vi "ShotLogSave.vi"(10 "Experiment State":T1={"error"={"status"=FALSE, "code"=0, "source"=""}, "Digitizer DAQmx Tasks"={"TaskArray"=[]}, "Digitizer Settings"={"Channel Settings"=[], "Card Settings"=[]}, "Synchronization Settings"={"Synchronizer"="PXI1Slot2", "source terminal"="GlobalSoftwareTrigger"}, "Digitizer Data"=[], "Next Shot#"="0", "System Message"="", "User Shot Notes"="", "Timing Settings"={"Timing Card Settings"=[], "Timing Channel Settings"=[[{"Delay (s)"=2.559999942779541, "Pulse width (s)"=0.009999999776482582, "Active"=TRUE, "Channel Name"="Fiber 8", "counter"="PXI1Slot8/ctr7"}]]}, "Timing Tasks"={"TaskArray"=[]}} {"Timing Settings"."Timing Channel Settings"."Pulse width (s)" format="%.3p"; "Timing Settings"."Timing Channel Settings"."Delay (s)" format="%.3p"; "Digitizer Settings"."Card Settings"."Global Edge Type" items=["Rising"=10280, "Falling"=10171]; "Digitizer Settings"."Card Settings"."Sample Rate" format="%#_3p"}) -> (2 "Experiment State":T1={"error"={"status"=FALSE, "code"=0, "source"=""}, "Digitizer DAQmx Tasks"={"TaskArray"=[]}, "Digitizer Settings"={"Channel Settings"=[], "Card Settings"=[]}, "Synchronization Settings"={"Synchronizer"="PXI1Slot2", "source terminal"="GlobalSoftwareTrigger"}, "Digitizer Data"=[], "Next Shot#"="0", "System Message"="", "User Shot Notes"="", "Timing Settings"={"Timing Card Settings"=[], "Timing Channel Settings"=[[{"Delay (s)"=2.559999942779541, "Pulse width (s)"=0.009999999776482582, "Active"=TRUE, "Channel Name"="Fiber 8", "counter"="PXI1Slot8/ctr7"}]]}, "Timing Tasks"={"TaskArray"=[]}} {"Timing Settings"."Timing Channel Settings"."Pulse width (s)" format="%.3p"; "Timing Settings"."Timing Channel Settings"."Delay (s)" format="%.3p"; "Digitizer Settings"."Card Settings"."Global Edge Type" items=["Rising"=10280, "Falling"=10171]; "Digitizer Settings"."Card Settings"."Sample Rate" format="%#_3p"})   [LabVIEW 2013]
uses:
  <vilib>/Utility/file.llb/Read From Spreadsheet File (string).vi
  <vilib>/Utility/NIReport.llb/NI_report.lvclass
  <vilib>/Utility/NIReport.llb/NI_ReportGenerationCore.lvlib
  <vilib>/printing/OpenHTMLReport.llb/Open HTML Report in Browser (Refnum).vi
  <vilib>/Utility/file.llb/Write To Spreadsheet File (string).vi
  <vilib>/Utility/NIReport.llb/Append Text Table to Report (wrap).vi
  Controls/ExperimentStateCluster.ctl
types:
  T1 = typedef "ExperimentStateCluster.ctl" = cluster{"error":errorcluster, "Digitizer DAQmx Tasks":cluster{"TaskArray":refnum<k21>[]}, "Digitizer Settings":cluster{"Channel Settings":cluster{"Channel":tag, "Channel Name":string, "Voltage Range":dbl, "Active":bool}[][], "Card Settings":cluster{"Start Time":dbl, "End Time":dbl, "Sample Rate":dbl, " Pre-Trigger Samples":u32, "Total Samples":i32, "Samples to Remove":u32, "Trigger Source":tag, "Global Edge Type":i32, "PXIStarLine":tag}[]}, "Synchronization Settings":cluster{"Synchronizer":refnum<k15>, "source terminal":string}, "Digitizer Data":waveform(dbl)[][], "Next Shot#":string, "System Message":string, "User Shot Notes":string, "Timing Settings":cluster{"Timing Card Settings":cluster{"Trigger Source":tag, "Clock Source":tag, "PXIStarLine":tag}[], "Timing Channel Settings":cluster{"Delay (s)":dbl, "Pulse width (s)":dbl, "Active":bool, "Channel Name":string, "counter":tag}[][]}, "Timing Tasks":cluster{"TaskArray":refnum<k21>[][]}}
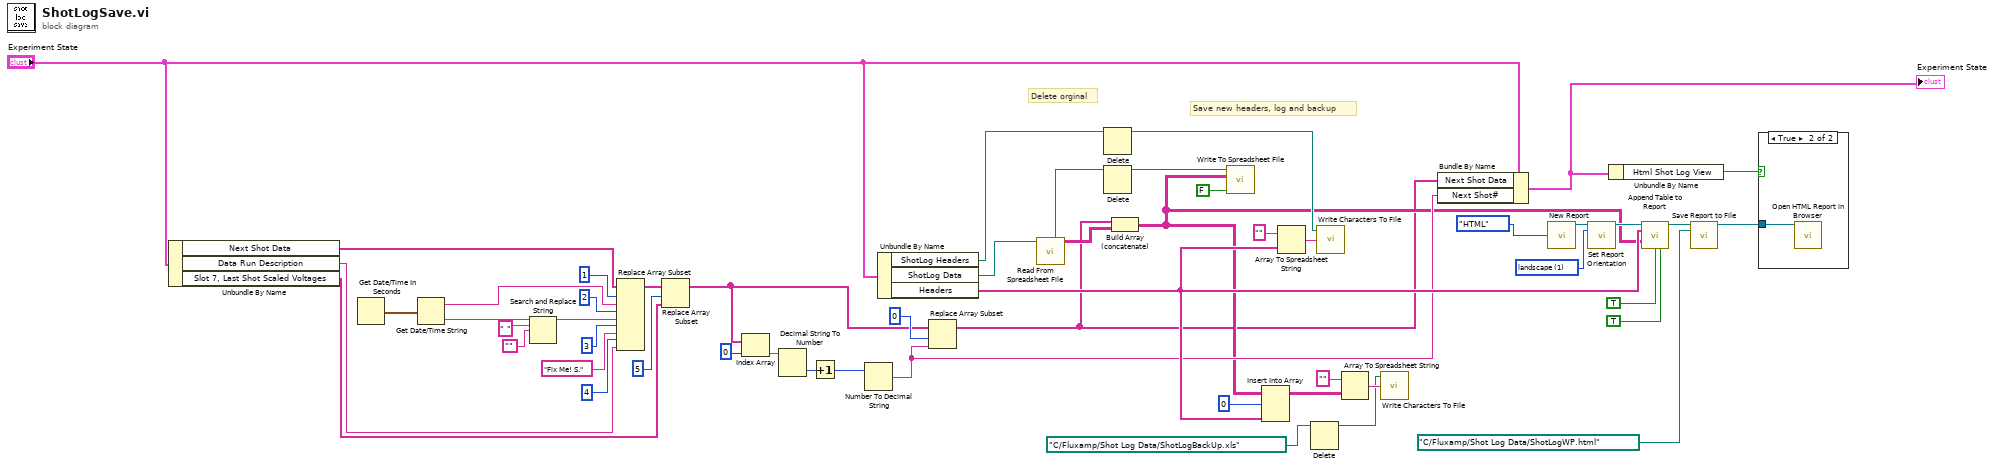
[diagram p0: block diagram]
diagram:
  w17 = u16 1 items=["portrait", "landscape"] ("orientation (portrait)")
  # "Delete orginal"
  # "Save new headers, log and backup"
  n1 = Unbundle By Name("Experiment State") -> ("Next Shot Data"=w50:string[], "Data Run Description"=w51:string, "Slot 7, Last Shot Scaled Voltages"=w52:string[])
  n2 = Get Date/Time In Seconds() -> (seconds since 1Jan1904=w47:timestamp)
  n3 = Get Date/Time String(seconds (now)=w47) -> (date string=w48:string, time string=w49:string)  [unwired: 2 out]
  n4 = Search and Replace String(input string=w49, search string=" ", replace string="") -> (result string=w34:string)  [unwired: 1 in, 7 out]
  n5 = Replace Array Subset(array=w50, new element #1=w48, index #1=1 ("index"), new element #2=w34, index #2=2 ("index"), new element #3="Fix Me! S." ("new element/subarray"), index #3=3 ("index"), new element #4=w51, index #4=4 ("index")) -> (w32:string[])
  n6 = Replace Array Subset(array=w32, new element=w52, index=5) -> (w9:string[])
  n7 = Index Array(array=w9, index=0 ("index (row)")) -> (element=w40:string)
  n8 = Decimal String To Number(string=w40) -> (number=w42:i32)  [unwired: 3 out]
  n9 = Increment(x=w42) -> (x+1=w41:i32)
  n10 = Number To Decimal String(number=w41) -> (decimal integer string=w11:string)  [unwired: 1 out]
  n11 = Unbundle By Name("Experiment State") -> ("ShotLog Headers"=w6:path, "ShotLog Data"=w8:path, "Headers"=w15:string[])
  n12 = Replace Array Subset(array=w9, new element=w11, index=0) -> (w1:string[])
  n13 = call-poly <vilib>:"Read From Spreadsheet File.vi"("file path (dialog if empty)"=w8) -> ("all rows"=w10:string[][], "new file path (Not A Path if cancelled)"=w7:path)  [unwired: 3 in, 6 out]
  n14 = Delete(path (use dialog)=w6) -> (deleted path=w23:path)  [unwired: 1 in, 5 out]
  n15 = Delete(path (use dialog)=w7) -> (deleted path=w4:path)  [unwired: 1 in, 5 out]
  n16 = Build Array (concatenate)(w1, w10) -> (w2:string[][])
  n17 = call-poly <vilib>:"Write To Spreadsheet File.vi"("append to file? (new file:F)"=FALSE, "2D data"=w2, "file path (dialog if empty)"=w4) -> ()  [unwired: 3 in, 3 out]
  n18 = Insert Into Array(array=w2, index (row)=0, new element=w15) -> (w24:string[][])  [unwired: 1 in]
  n19 = Array To Spreadsheet String(array=w15, 3:"" ("format string")) -> (spreadsheet string=w29:string)  [unwired: 1 in]
  n20 = Delete(path (use dialog)=path "C:/Fluxamp/Shot Log Data/ShotLogBackUp.xls" ("file path (dialog if empty)")) -> (deleted path=w22:path)  [unwired: 1 in, 5 out]
  n21 = call <vilib>:"Write Characters To File.vi"("character string"=w29, "file path (dialog if empty)"=w23) -> ()  [unwired: 1 in, 3 out]
  n22 = Array To Spreadsheet String(array=w24, 3:"" ("format string")) -> (spreadsheet string=w26:string)  [unwired: 1 in]
  n23 = call <vilib>:"Write Characters To File.vi"("character string"=w26, "file path (dialog if empty)"=w22) -> ()  [unwired: 1 in, 3 out]
  n24 = Bundle By Name(cluster="Experiment State", "Next Shot Data"=w1, "Next Shot#"=w11) -> (w44:T1)
  "Experiment State" <- w44
  n25 = call <vilib>:"New Report.vi"("report type"=enum16{"Standard Report", "HTML"}."HTML") -> ("report out"=w18:refnum<class "NI_report.lvclass">)  [unwired: 13 in, 1 out]
  n26 = call-dynamic "Set Report Orientation.vi"("report in"=w18, "orientation (portrait)"=w17) -> ("report out"=w16:refnum<class "NI_report.lvclass">)  [unwired: 12 in, 1 out]
  n27 = Unbundle By Name(w44) -> ("Html Shot Log View"=w14:bool)
  n28 = call-poly <vilib>:"Append Table to Report.vi"("report in"=w16, "column headers"=w15, "text data"=w2, "separate page? (NO)"=TRUE ("separate page?"), "show grid lines (YES)"=TRUE ("show grid lines")) -> ("report out"=w13:refnum<class "NI_report.lvclass">)  [unwired: 7 in, 3 out]
  n29 = call-dynamic "Save Report to File.vi"("report in"=w13, "report file path"=path "C:/Fluxamp/Shot Log Data/ShotLogWP.html" ("file path (dialog if empty)")) -> ("report out"=w12:refnum<class "NI_report.lvclass">)  [unwired: 12 in, 1 out]
  n30 = case shown="True" w14 {
    tunnel: w12 -> [_ w54]
    frame False {
    }
    frame True {
      n31 = call-poly <vilib>:"Open HTML Report in Browser.vi"("report in"=w54) -> ()  [unwired: 12 in, 3 out]
    }
  }
